vi "Start and Stop Test Example.vi"() -> ()   [LabVIEW 2020]
uses:
  FlexLoggerTagHelpers.lvlib
panel:
  in  "Stop":bool
  out "Elapsed Time (s)":dbl
  in  "test time (s)":dbl=60.0 caption="Time Target (s)"
  out "IsTestSessionRunning":bool
  out "Last Test Start Time":timestamp
  # "Overview: This example demonstrates using the FlexLogger test running tag (IsTestSessionRunning) to start a test on the currently open FlexLogger project for one minute and then stop the test. \nRequirements: LabVIEW Full Development System, FlexLogger\nInstructions:\n1. Launch FlexLogger\n     a. Create a Project\n     b. Configure one or more channels in the Channel Specification\n     c. Using the Project >> Settings menu, enable Publish SystemLink Tags (Export) and Consume SystemLink Tags (Import)\n     d. Restart the FlexLogger Project\n2. Set the desired testing duration on this VI and run this VI.\n3. The IsTestSessionRunning tag value will be read and displayed on the front panel until the test time has elapsed."
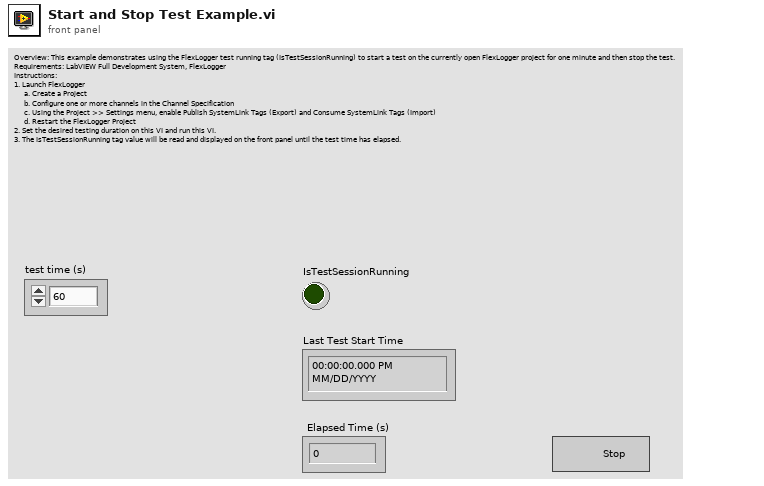
[diagram p1: front panel]
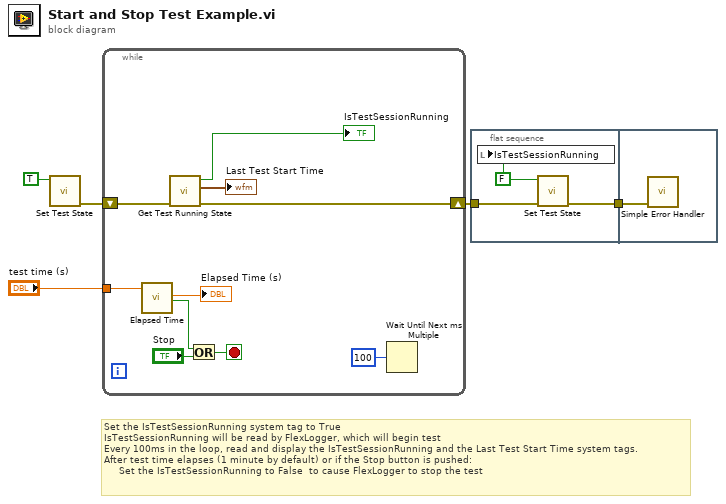
[diagram p0: block diagram]
diagram:
  # "Set the IsTestSessionRunning system tag to True\nIsTestSessionRunning will be read by FlexLogger, which will begin test\nEvery 100ms in the loop, read and display the IsTestSessionRunning and the Last Test Start Time system tags.\nAfter test time elapses (1 minute by default) or if the Stop button is pushed:\n     Set the IsTestSessionRunning to False  to cause FlexLogger to stop the test"
  n1 = call "Set Test State.vi"("IsTestRunning"=TRUE ("Logging?")) -> ("error out"=w4:errorcluster)  [unwired: 10 in]
  n2 = while {
    shift-right: [w15] -> w2
    shift-left: w4 -> [w14]
    tunnel: "test time (s)" -> [w11]
    stop <- w6 stop-if-true
    n3 = call "Elapsed Time"("Time Target (s)"=w11) -> ("Elapsed Time (s)"=→"Elapsed Time (s)":dbl, "Time has Elapsed"=w8:bool)  [unwired: 11 in, 6 out]
    n4 = call "Get Test Running State.vi"("error in (no error)"=w14) -> ("error out"=w15:errorcluster, "Last Test Start Time"=→"Last Test Start Time":timestamp, "Is Test Running"=→"IsTestSessionRunning":bool)  [unwired: 8 in]
    n5 = Or(x=w8, y="Stop") -> (x .or. y?=w6:bool)
    n6 = Wait Until Next ms Multiple(millisecond multiple=u32 100 ("milliseconds to wait")) -> ()  [unwired: 1 out]
  }
  n7 = flat-sequence {
    tunnel: w2 -> [w18]
    tunnel: [w17] -> w1
    tunnel: w1 -> [w19]
    frame #0 {
      w16 = FALSE ("Logging?")
      n8 = local write "IsTestSessionRunning"(w16) -> ()
      n9 = call "Set Test State.vi"("error in"=w18, "IsTestRunning"=w16) -> ("error out"=w17:errorcluster)  [unwired: 9 in]
    }
    frame #1 {
      n10 = call <vilib>:"Simple Error Handler.vi"("error in (no error)"=w19) -> ()  [unwired: 4 in, 5 out]
    }
  }
